vi "Read Session Log.vi"(8 "error in (no error)":errorcluster, 11 "DAQ Device in":refnum<class "DAQ Device.lvclass">) -> (0 "error out":errorcluster, 2 "Session Handle":T1, 3 "DAQ Device out":refnum<class "DAQ Device.lvclass">)   [LabVIEW 2014, in "DAQ Device.lvclass"]
uses:
  DAQ Device.lvclass
  <userlib>/_Session Fwk/Typedefs/Session Handle.ctl
  <userlib>/_Session Fwk/Session - Root.lvclass
  DAQ Device.lvclass/DAQ Device.ctl
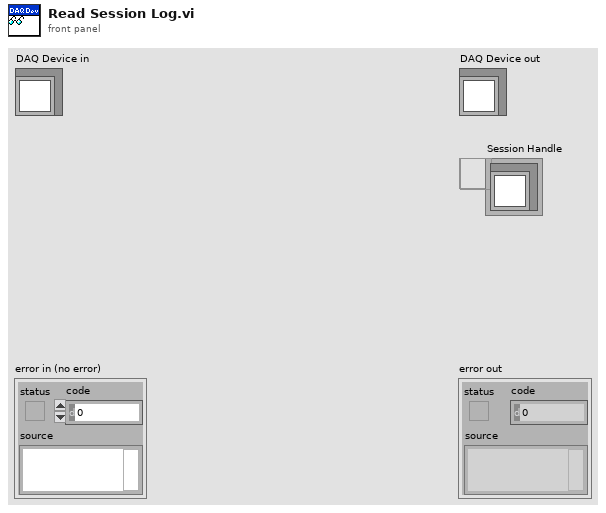
[diagram p1: front panel]
types:
  T1 = typedef "Session - Root.lvclass/Session Handle.ctl" = refnum<data-value>
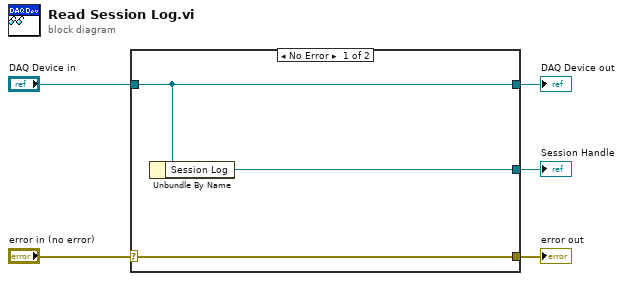
[diagram p0: block diagram]
diagram:
  n1 = case shown="No Error" "error in (no error)" {
    selector: "error in (no error)" -> [w8 w9]
    tunnel: [w8 w9] -> w4
    tunnel: [w7 w10] -> w2
    tunnel: "DAQ Device in" -> [w7 w10]
    tunnel: [w6 _] -> w1
    frame No Error {
      n2 = Unbundle By Name(w7) -> ("Session Log"=w6:T1)
    }
    frame Error {
    }
  }
  "error out" <- w4
  "DAQ Device out" <- w2
  "Session Handle" <- w1
